vi "electrical measurements MR16.vi"() -> ()   [LabVIEW 2011]
doc: "This example illustrates how to use autosetup and acquire multiple waveforms from several channels using the following steps:\n\n1. Specify a valid VISA session. \n2. Specify Channel A. \n3. Specify Channel B.\n4. Specify a time-out value for reading waveform.\n5. Run the VI. The graph displays waveforms you acquire."
uses:
  <instrlib>/Tektronix DPO MSO 2000 4000 Series/Public/Configure/Configure Trigger (Edge).vi
  <instrlib>/Tektronix DPO MSO 2000 4000 Series/Public/Data/Read (Multiple Waveforms).vi
  <instrlib>/Tektronix DPO MSO 2000 4000 Series/Tektronix DPO MSO 2000 4000 Series.lvlib
panel:
  in  "Channel C(2: Channel 3)":u16(ring) items=["Channel 1", "Channel 2", "Channel 3", "Channel 4", "Math", "Reference 1", "Reference 2", "Reference 3", "Reference 4", "Bus 1", "Bus 2"]
  in  "Vertical Coupling (1: DC)":u16(ring)=1 items=["AC", "DC", "Ground"]
  in  "Vertical Coupling (1: DC)":u16(ring)=1 items=["AC", "DC", "Ground"]
  in  "Maximum Time (20000ms)":u32=20000
  in  "Channel B (1: Channel 2)":u16(ring)=1 items=["Channel 1", "Channel 2", "Channel 3", "Channel 4", "Math", "Reference 1", "Reference 2", "Reference 3", "Reference 4"]
  in  "Channel A (0: Channel 1)":u16(ring) items=["Channel 1", "Channel 2", "Channel 3", "Channel 4", "Math", "Reference 1", "Reference 2", "Reference 3", "Reference 4"]
  in  "VISA Resource Name":refnum<visa-resource-name>
  out "Waveform Graph":waveform(dbl)[](graph)
  # "(c) 2006 - 2012. National Instruments Corporation. ALL RIGHTS RESERVED."
  # "Channel A"
  # "Channel B"
  # "Channel C"
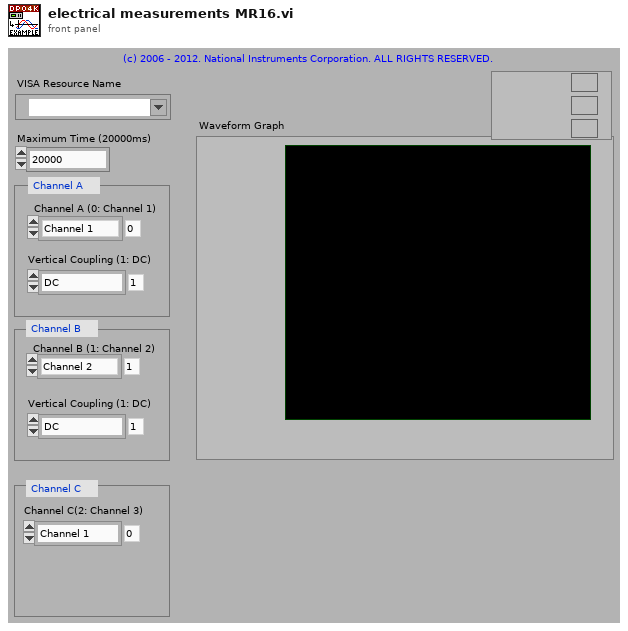
[diagram p1: front panel]
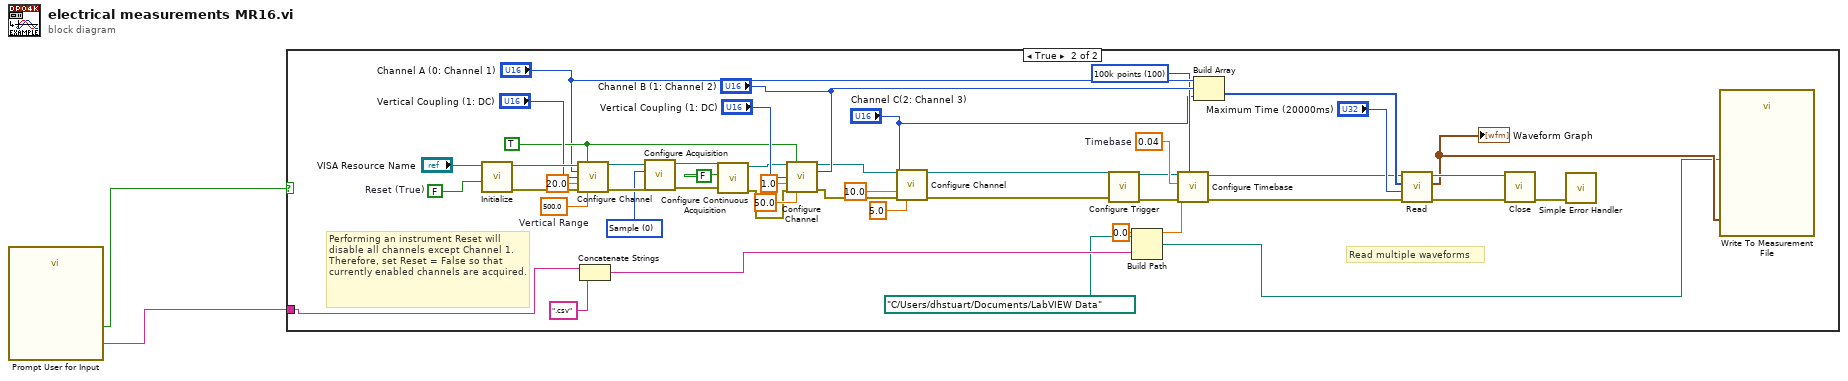
[diagram p0: block diagram]
diagram:
  n1 = call "Prompt User for Input"() -> ("file_name"=w1:string, "OK"=w2:bool)  [unwired: 17 in, 1 out]
  n2 = case shown="True" w2 {
    tunnel: w1 -> [_ w25]
    frame False {
    }
    frame True {
      w10 = u16 0 items=["Sample", "Peak Detect", "Hi Res", "Envelope", "Average"] ("Acquisition Type (0: Sample)")
      w26 = u32 100 items=["1000 points"=1, "10k points"=10, "100k points"=100, "1M points"=1000, "5M points"=5000, "10M points"=10000] ("Record Length (10: 10k points)")
      w35 = 0.04  # Timebase
      w30 = 500.0  # Vertical Range
      w34 = TRUE ("Enable Channel (T: Enable)")
      w42 = FALSE  # Reset (True)
      # "Performing an instrument Reset will disable all channels except Channel 1. Therefore, set Reset = False so that currently enabled channels are acquired."
      # "Read multiple waveforms"
      n3 = call <instrlib>:"Initialize.vi"("Reset (True)"=w42, "VISA resource name"="VISA Resource Name") -> ("error out"=w40:errorcluster, "VISA resource name out"=w41:refnum<visa-resource-name>)  [unwired: 8 in]
      n4 = call <instrlib>:"Configure Channel.vi"("VISA resource name"=w41, "Enable Channel (T: Enable)"=w34, "Channel (0: Channel 1)"="Channel A (0: Channel 1)", "Vertical Coupling (1: DC)"="Vertical Coupling (1: DC)", "Probe Attenuation (1)"=20.0, "error in (no error)"=w40, "Vertical Range (10.0 V)"=w30) -> ("VISA resource name out"=w14:refnum<visa-resource-name>, "error out"=w12:errorcluster)  [unwired: 7 in]
      n5 = Concatenate Strings(w25, ".csv" ("string")) -> (w23:string)
      n6 = call <instrlib>:"Configure Acquisition.vi"("error in (no error)"=w12, "Acquisition Type (0: Sample)"=w10, "VISA resource name"=w14) -> ("error out"=w11:errorcluster, "VISA resource name out"=w13:refnum<visa-resource-name>)  [unwired: 7 in]
      n7 = call <instrlib>:"Configure Continuous Acquisition.vi"("error in (no error)"=w11, "Enable Continuous Acquisition Mode (T: Enable)"=FALSE, "VISA resource name"=w13) -> ("error out"=w16:errorcluster, "VISA resource name out"=w17:refnum<visa-resource-name>)  [unwired: 7 in]
      n8 = call <instrlib>:"Configure Channel.vi"("VISA resource name"=w17, "Enable Channel (T: Enable)"=w34, "Channel (0: Channel 1)"="Channel B (1: Channel 2)", "Vertical Coupling (1: DC)"="Vertical Coupling (1: DC)", "Probe Attenuation (1)"=1.0, "error in (no error)"=w16, "Vertical Range (10.0 V)"=50.0) -> ("VISA resource name out"=w9:refnum<visa-resource-name>, "error out"=w8:errorcluster)  [unwired: 7 in]
      n9 = call <instrlib>:"Configure Channel.vi"("VISA resource name"=w9, "Channel (0: Channel 1)"="Channel C(2: Channel 3)", "Probe Attenuation (1)"=10.0, "error in (no error)"=w8, "Vertical Range (10.0 V)"=5.0) -> ("VISA resource name out"=w7:refnum<visa-resource-name>, "error out"=w6:errorcluster)  [unwired: 9 in]
      n10 = call-poly <instrlib>:"Configure Trigger.vi"("VISA resource name"=w7, "error in (no error)"=w6) -> ("VISA resource name out"=w20:refnum<visa-resource-name>, "error out"=w19:errorcluster)  [unwired: 12 in]
      n11 = Build Path(base path=path "C:/Users/dhstuart/Documents/LabVIEW Data", name or relative path=w23) -> (appended path=w21:path)
      n12 = call <instrlib>:"Configure Timebase.vi"("Record Length (10: 10k points)"=w26, "error in (no error)"=w19, "Position (10 %)"=0.0, "Timebase (0.0005 s)"=w35, "VISA resource name"=w20) -> ("error out"=w36:errorcluster, "VISA resource name out"=w37:refnum<visa-resource-name>)  [unwired: 5 in]
      n13 = Build Array("Channel A (0: Channel 1)", "Channel B (1: Channel 2)", "Channel C(2: Channel 3)") -> (w47:u16[])
      n14 = call-poly <instrlib>:"Read.vi"("error in (no error)"=w36, "Maximum Time (10000ms)"="Maximum Time (20000ms)", "Channels"=w47, "VISA resource name"=w37) -> ("error out"=w45:errorcluster, "Waveform Data"=w31:waveform(dbl)[], "VISA resource name out"=w46:refnum<visa-resource-name>)  [unwired: 5 in]
      "Waveform Graph" <- w31
      n15 = call <instrlib>:"Close.vi"("error in (no error)"=w45, "VISA resource name"=w46) -> ("error out"=w44:errorcluster)  [unwired: 9 in]
      n16 = call <vilib>:"Simple Error Handler.vi"("error in (no error)"=w44) -> ()  [unwired: 4 in, 5 out]
      n17 = call "Write To Measurement File"("Signals"=w31, "Filename"=w21) -> ()  [unwired: 15 in, 3 out]
    }
  }
